vi "Cache-Find.vi"(7 "Idx":i32, 8 "error in":errorcluster, 9 "Serial":string, 10 "Variant":string) -> (0 "error out":errorcluster, 1 "ProductComponent":T1, 2 "Result":T2, 3 "Found":bool)   [LabVIEW 2016]
doc: "Go to DB->WriteStationValues action\nReturn boolean flag to show if data was saved to DB successfully\n\nWabco 2017 All right reserved\nAuthor: maciej.szupienko@wabco-auto.com"
uses:
  Cache.TestSteps.Fglb.ResultData.ctl
  Database/ProdaNG/Controls/ProdaNG.ProcessResult.ctl
  Database/ProdaNG/Controls/ProdaNG.ProcessStepResult.ctl
  Database/ProdaNG/Controls/ProdaNG.TestStepResult.ctl
  Database/ProdaNG/Controls/ProdaNG.TestValueResult.ctl
  Database/ProdaNG/Controls/ProdaNG.ProductComponent.ctl
  Cache.Action.ctl
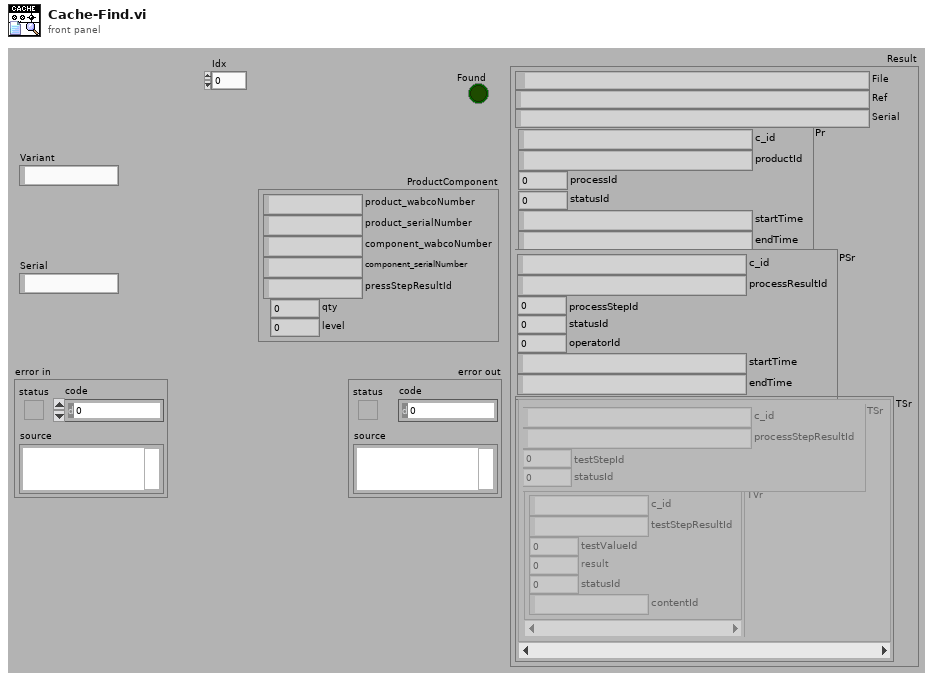
[diagram p1: front panel]
types:
  T1 = typedef "ProdaNG.ProductComponent.ctl" = cluster{"product_wabcoNumber":string, "product_serialNumber":string, "component_wabcoNumber":string, "component_serialNumber":string, "pressStepResultId":string, "qty":i32, "level":i32}
  T2 = typedef "Cache.TestSteps.Fglb.ResultData.ctl" = cluster{"File":path, "Ref":string, "Serial":string, "Pr":T3, "PSr":T4, "TSr":cluster{"TSr":T5, "TVr":T6[]}[]}
  T3 = typedef "ProdaNG.ProcessResult.ctl" = cluster{"c_id":string, "productId":string, "processId":i32, "statusId":i32, "startTime":string, "endTime":string}
  T4 = typedef "ProdaNG.ProcessStepResult.ctl" = cluster{"c_id":string, "processResultId":string, "processStepId":i32, "statusId":i32, "operatorId":i32, "startTime":string, "endTime":string}
  T5 = typedef "ProdaNG.TestStepResult.ctl" = cluster{"c_id":string, "processStepResultId":string, "testStepId":i32, "statusId":i32}
  T6 = typedef "ProdaNG.TestValueResult.ctl" = cluster{"c_id":string, "testStepResultId":string, "testValueId":i32, "result":dbl, "statusId":i32, "contentId":string}
  T7 = typedef "Cache.Action.ctl" = enum32{"idle", "constructor", "destructor", "--- Cache ---", "Find", "FindToExport", "Move", "Delete"}
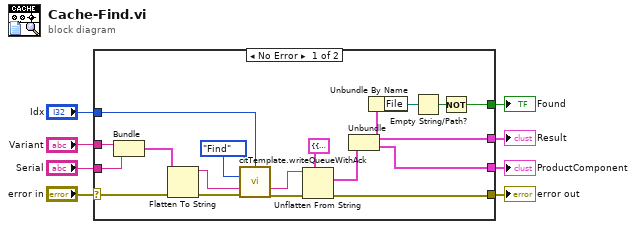
[diagram p0: block diagram]
diagram:
  n1 = case shown="No Error" "error in" {
    selector: "error in" -> [w13 _]
    tunnel: "Idx" -> [w26 _]
    tunnel: [w21 _] -> w7
    tunnel: [w12 _] -> w5
    tunnel: [w20 _] -> w4
    tunnel: "Variant" -> [w18 _]
    tunnel: "Serial" -> [w17 _]
    tunnel: [w9 _] -> w1
    frame No Error {
      n2 = Bundle("Variant"=w18, "Serial"=w17) -> (w14:cluster{"Variant":string, "Serial":string})  [unwired: 1 in]
      n3 = Flatten To String(anything=w14, error in (no error)=w13) -> (data string=w15:string, error out=w16:errorcluster)  [unwired: 2 in, 1 out]
      n4 = call "citTemplate.writeQueueWithAck.vi"("instance (0)"=w26, "event in"=Cache.Action."Find" ("Action"), "(flatten) data in"=w15, "error in (no error)"=w16) -> ("notification data"=w24:string, "error out"=w25:errorcluster)  [unwired: 9 in, 1 out]
      n5 = Unflatten From String(type=cluster{"Result":T2, "ProductComponent":T1} {"Result"={"File"=path "", "Ref"="", "Serial"="", "Pr"={"c_id"="", "productId"="", "processId"=0, "statusId"=0, "startTime"="", "endTime"=""}, "PSr"={"c_id"="", "processResultId"="", "processStepId"=0, "statusId"=0, "operatorId"=0, "startTime"="", "endTime"=""}, "TSr"=[]}, "ProductComponent"={"product_wabcoNumber"="", "product_serialNumber"="", "component_wabcoNumber"="", "component_serialNumber"="", "pressStepResultId"="", "qty"=0, "level"=0}} ("output cluster"), binary string=w24, error in (no error)=w25) -> (value=w22:cluster{"Result":T2, "ProductComponent":T1}, error out=w21:errorcluster)  [unwired: 2 in, 1 out]
      n6 = Unbundle(w22) -> ("Result"=w12:T2, "ProductComponent"=w20:T1)
      n7 = Unbundle By Name(w12) -> ("File"=w11:path)
      n8 = Empty String/Path?(string/path=w11) -> (empty?=w10:bool)
      n9 = Not(x=w10) -> (.not. x?=w9:bool)
    }
    frame Error {
    }
  }
  "error out" <- w7
  "Result" <- w5
  "ProductComponent" <- w4
  "Found" <- w1
